vi "SaveMeasurements.vi"(7 "Sample name":string, 8 "error in (no error)":errorcluster, 9 "Type":string, 10 "Text":string, 11 "Path":path) -> (0 "error out":errorcluster)   [LabVIEW 2014]
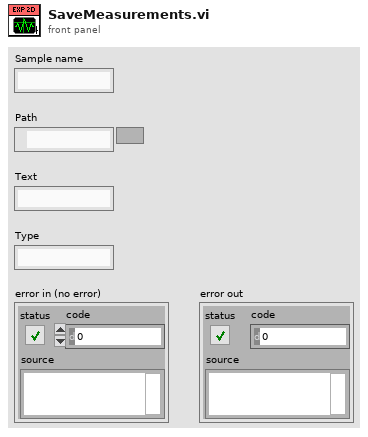
[diagram p1: front panel]
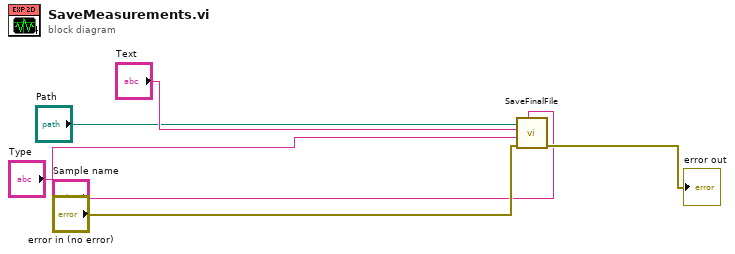
[diagram p0: block diagram]
diagram:
  n1 = call "SaveFinalFile.vi"("Sample name"="Sample name", "error in (no error)"="error in (no error)", "Type"="Type", "Text"="Text", "Path"="Path") -> ("error out"=→"error out":errorcluster)  [unwired: 6 in]
